vi "remove tag.vi"(8 "error in":errorcluster, 10 "tag":refnum<class "data bus tag description.lvclass">, 11 "tag collection in":refnum<class "data bus tag collection.lvclass">) -> (0 "error out":errorcluster, 1 "removed tag":refnum<class "data bus tag description.lvclass">, 3 "tag collection out":refnum<class "data bus tag collection.lvclass">)   [LabVIEW 2013, in "data bus tag collection.lvclass"]
uses:
  data bus tag collection.lvclass
  tag/data bus tag description.lvclass
  tag/data bus tag description.lvclass/data bus tag description.ctl
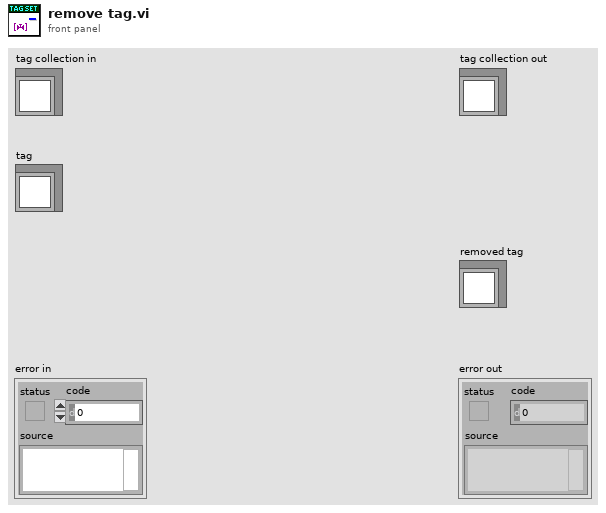
[diagram p1: front panel]
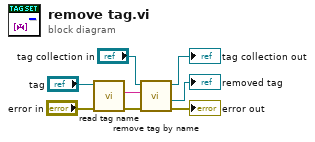
[diagram p0: block diagram]
diagram:
  n1 = call "read tag name.vi"("error in"="error in", "system tag in"="tag") -> ("error out"=w5:errorcluster, "name"=w2:string)  [unwired: 7 in, 1 out]
  n2 = call "remove tag by name.vi"("error in"=w5, "tag"=w2, "tag collection in"="tag collection in") -> ("error out"=→"error out":errorcluster, "removed tag"=→"removed tag":refnum<class "data bus tag description.lvclass">, "tag collection out"=→"tag collection out":refnum<class "data bus tag collection.lvclass">)  [unwired: 6 in]
